vi "Read Buffer By Name.vi"(8 "error in (no error)":errorcluster, 10 "Name":string, 11 "BufferMap in":refnum<data-value>) -> (0 "error out":errorcluster, 1 "found":bool, 2 "Buffer":refnum<data-value>, 3 "BufferMap":refnum<data-value>)   [LabVIEW 2013, in "VariantBufferMap.lvclass"]
uses:
  VariantBufferMap.lvclass
  VariantBuffer/VariantBuffer.lvclass
  VariantBufferMap.lvclass/VariantBufferMap.ctl
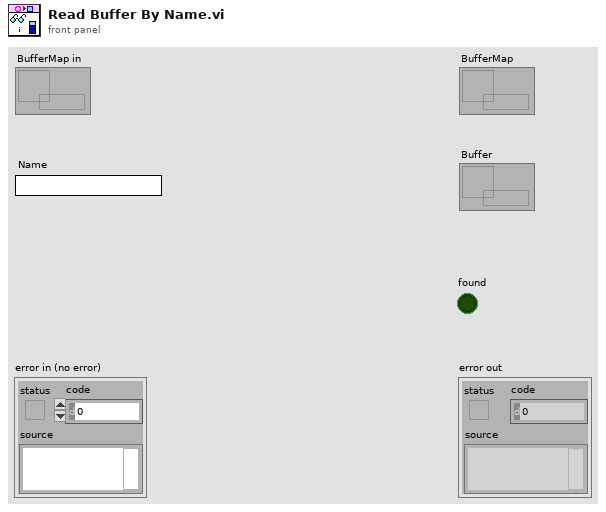
[diagram p1: front panel]
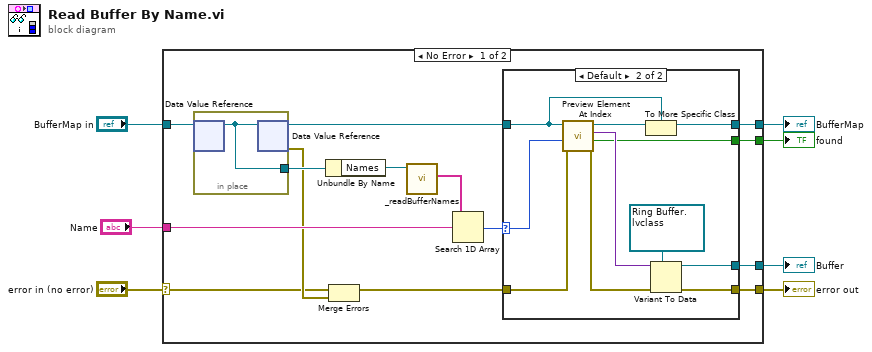
[diagram p0: block diagram]
diagram:
  n1 = case shown="No Error" "error in (no error)" {
    selector: "error in (no error)" -> [w9 w36]
    tunnel: [w20 w37] -> w5
    tunnel: "BufferMap in" -> [w16 w37]
    tunnel: [w18 _] -> w4
    tunnel: [w17 _] -> w3
    tunnel: "Name" -> [w13 _]
    tunnel: [w11 w36] -> w1
    frame No Error {
      n2 = in-place {
        in-place-border: [w35] -> w21
        n3 = in-place-dvr #1(w16) -> (w35:refnum<class "VariantBufferMap.lvclass">)  [unwired: 1 out]
        n4 = in-place-dvr #1(w35) -> (w15:refnum<data-value>, w10:errorcluster)
      }
      n5 = Unbundle By Name(w21) -> ("Names"=w19:refnum<data-value>)
      n6 = Merge Errors(w9, w10) -> (w8:errorcluster)
      n7 = call "_readBufferNames.vi"("Data Value Reference in"=w19) -> ("Names"=w14:string[])  [unwired: 9 in, 1 out]
      n8 = Search 1D Array(1D array=w14, element=w13) -> (index of element=w12:i32)  [unwired: 1 in]
      n9 = case shown="Default" w12 {
        selector: w12 -> [_ w28]
        tunnel: [w23 w34] -> w20
        tunnel: [_ w30] -> w18
        tunnel: [_ w29] -> w17
        tunnel: w15 -> [w23 w27]
        tunnel: [w22 w25] -> w11
        tunnel: w8 -> [w22 w24]
        frame -1 {
        }
        frame Default {
          n10 = call "Preview Element At Index.vi"("error in"=w24, "index (-1: last)"=w28, "Buffer in"=w27) -> ("error out"=w26:errorcluster, "found"=w29:bool, "element"=w32:variant, "Buffer"=w33:refnum<data-value>)  [unwired: 5 in]
          n11 = To More Specific Class(target class=w27, reference=w33) -> (specific class reference=w34:refnum<data-value>)  [unwired: 1 in, 1 out]
          n12 = Variant To Data(error in=w26, type=refnum<data-value> refnum ("Buffer"), Variant=w32) -> (data=w30:refnum<data-value>, error out=w25:errorcluster)
        }
      }
    }
    frame Error {
    }
  }
  "error out" <- w1
  "BufferMap" <- w5
  "Buffer" <- w4
  "found" <- w3
